vi "Log State.vi"(8 "error in (no error)":errorcluster, 10 "Model Status":T3, 11 "Data":T1) -> (0 "error out":errorcluster, 3 "Data out":T1)   [LabVIEW 2014, in "Logger.lvlib"]
uses:
  Logger.lvlib
  Model/TypeDefs/Get Model Status Control.ctl
  Model/Model.lvlib
  TypeDefs/Logger State.ctl
  TypeDefs/Logger Data.ctl
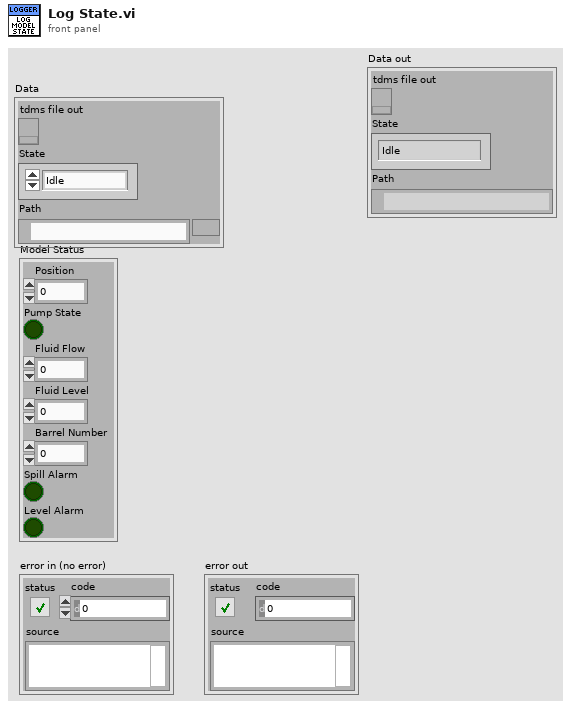
[diagram p1: front panel]
types:
  T1 = typedef "Logger.lvlib/Logger Data.ctl" = cluster{"tdms file out":refnum<k34>, "State":T2, "Path":path}
  T2 = typedef "Logger.lvlib/Logger State.ctl" = enum16{"Idle", "Working"}
  T3 = typedef "Model.lvlib/Get Model Status Control.ctl" = cluster{"Position":dbl, "Pump State":bool, "Fluid Flow":dbl, "Fluid Level":dbl, "Barrel Number":i32, "Spill Alarm":bool, "Level Alarm":bool}
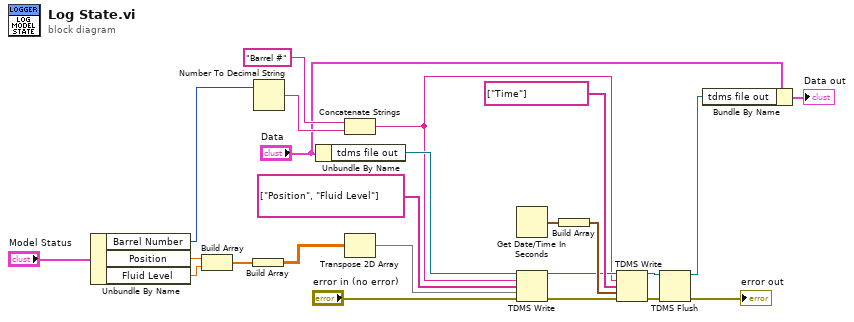
[diagram p0: block diagram]
diagram:
  n1 = Unbundle By Name("Model Status") -> ("Barrel Number"=w7:i32, "Position"=w12:dbl, "Fluid Level"=w13:dbl)
  n2 = Build Array(w12, w13) -> (w19:dbl[])
  n3 = Build Array(w19) -> (w20:dbl[][])
  n4 = Number To Decimal String(number=w7) -> (decimal integer string=w5:string)  [unwired: 1 in]
  n5 = Unbundle By Name("Data") -> ("tdms file out"=w10:refnum<k34>)
  n6 = Concatenate Strings("Barrel #", w5) -> (w4:string)
  n7 = Transpose 2D Array(2D array=w20) -> (transposed array=w21:dbl[][])
  n8 = Get Date/Time In Seconds() -> (seconds since 1Jan1904=w17:timestamp)
  n9 = TDMS Write(0:w10, 5:w4, 7:string[] ["Position", "Fluid Level"], 9:w21, 11:"error in (no error)") -> (4:w15:refnum<k34>, 15:w14:errorcluster)  [unwired: 1 in, 2 out]
  n10 = Build Array(w17) -> (w18:timestamp[])
  n11 = TDMS Write(0:w15, 5:w4, 7:string[] ["Time"], 9:w18, 11:w14) -> (4:w23:refnum<k34>, 15:w22:errorcluster)  [unwired: 1 in, 2 out]
  n12 = TDMS Flush(4:w22, 7:w23) -> (0:→"error out":errorcluster, 3:w1:refnum<k34>)
  n13 = Bundle By Name(cluster="Data", "tdms file out"=w1) -> (→"Data out":T1)
